vi "add_text_field.vi"(8 "error in":errorcluster, 9 "field_value":string, 10 "field_name":string, 11 "MultipartForm in":refnum<class "MultipartForm.lvclass">) -> (0 "error out":errorcluster, 2 "success":bool, 3 "MultipartForm out":refnum<class "MultipartForm.lvclass">)   [LabVIEW 2020, in "reqwest.lvlib" / "MultipartForm.lvclass"]
uses:
  MultipartForm.lvclass
  MultipartForm.lvclass/MultipartForm.ctl
  lv_reqwest_64.dll
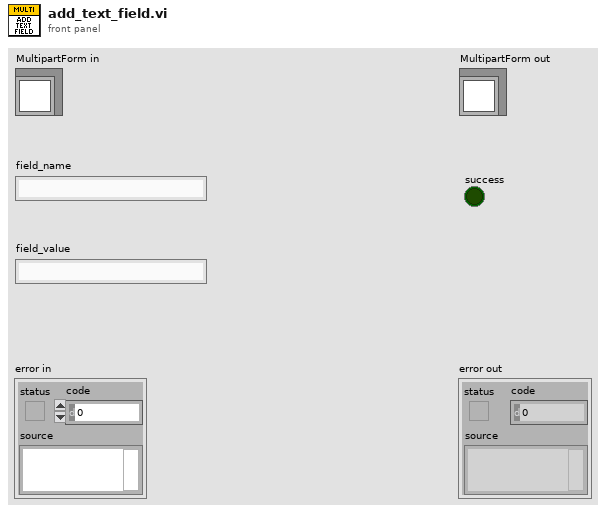
[diagram p1: front panel]
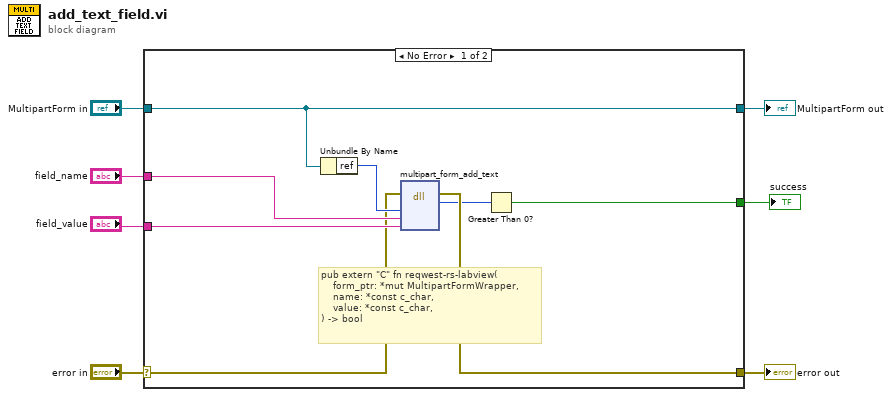
[diagram p0: block diagram]
diagram:
  n1 = case shown="No Error" "error in" {
    selector: "error in" -> [w11 w17]
    tunnel: [w10 w17] -> w6
    tunnel: [w15 w16] -> w4
    tunnel: "MultipartForm in" -> [w15 w16]
    tunnel: "field_name" -> [w13 _]
    tunnel: "field_value" -> [w12 _]
    tunnel: [w8 _] -> w1
    frame No Error {
      # "pub extern \"C\" fn reqwest-rs-labview(\n    form_ptr: *mut MultipartFormWrapper,\n    name: *const c_char,\n    value: *const c_char,\n) -> bool"
      n2 = Unbundle By Name(w15) -> ("ref"=w14:u64)
      n3 = dll-call lib="C:/Projects/reqwest-rs-labview/lv_src/lv_reqwest_*.*" fn="multipart_form_add_text"(error in=w11, "form"=w14, "field_name"=w13, "field_value"=w12) -> (error out=w10:errorcluster, "bool"=w9:u8)  [unwired: 5 in, 1 out]
      n4 = Greater Than 0?(x=w9) -> (x > 0?=w8:bool)
    }
    frame Error {
    }
  }
  "error out" <- w6
  "MultipartForm out" <- w4
  "success" <- w1
